vi "ExpandXi.vi"(2 "N":i32=1024, 3 "X":dbl[](array[numeric])) -> (1 "X 2":dbl[](array[numeric]))   [LabVIEW 2020]
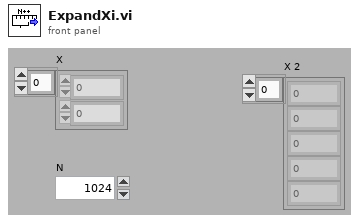
[diagram p1: front panel]
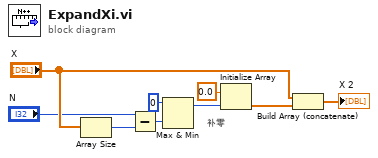
[diagram p0: block diagram]
diagram:
  # "补零"
  n1 = Array Size(array="X") -> (size(s)=w5:i32)
  n2 = Subtract(x="N", y=w5) -> (x-y=w1:i32)
  n3 = Max & Min(x=0, y=w1) -> (max(x,y)=w6:i32)  [unwired: 1 out]
  n4 = Initialize Array(0.0, w6) -> (w8:dbl[])
  n5 = Build Array (concatenate)("X", w8) -> (→"X 2":dbl[])
